vi "S4GUI.vi"(7 "Tab ObsEng":enum32{"Obs", "CCD modes", "Guider", "Eng"}(tab)) -> ()   [LabVIEW 2018] (continued)
            n4203 = call "Read WPROT.vi"("error in (no error)"=w9679, "Instrument in"=w9681) -> ("error out"=w9674:errorcluster, "Opt_Selector.lvclass"=w9677:refnum<class "Opt_Selector.lvclass">, "Instrument out"=w9682:refnum<class "Instrument.lvclass">)  [unwired: 7 in]
            n4204 = call-dynamic "Read sequencia_ant.vi"("error in (no error)"=w9674, "Opt_Selector in"=w9677) -> ("error out"=w9673:errorcluster, "sequencia_ant"=w9675:u16, "Opt_Selector out"=w9676:refnum<class "Opt_Selector.lvclass">)  [unwired: 7 in]
            n4205 = call-dynamic "Write sequencia.vi"("error in (no error)"=w9673, "sequencia"=w9675, "Opt_Selector in"=w9676) -> ("error out"=w9668:errorcluster, "Opt_Selector out"=w9669:refnum<class "Opt_Selector.lvclass">)  [unwired: 7 in]
            n4206 = call-dynamic "Read State Machine.vi"("error in (no error)"=w9668, "Device in"=w9669) -> ("error out"=w9671:errorcluster, "State Machine.lvclass"=w9666:refnum<class "State Machine.lvclass">, "Device out"=w9667:refnum<class "Opt_Selector.lvclass">)  [unwired: 7 in]
            n4207 = call "Next State.vi"("error in (no error)"=w9671, "New_State"=10, "State Machine in"=w9666) -> ("error out"=w9670:errorcluster, "State Machine out"=w9665:refnum<class "State Machine.lvclass">)  [unwired: 7 in]
            n4208 = call-dynamic "Write State Machine.vi"("error in (no error)"=w9670, "State Machine.lvclass"=w9665, "Device in"=w9667) -> ("error out"=w9664:errorcluster, "Device out"=w9663:refnum<class "Opt_Selector.lvclass">)  [unwired: 7 in]
            n4209 = call "Write WPROT.vi"("error in (no error)"=w9664, "Opt_Selector.lvclass"=w9663, "Instrument in"=w9682) -> ("error out"=w9661:errorcluster, "Instrument out"=w9662:refnum<class "Instrument.lvclass">)  [unwired: 7 in]
            n4210 = call "Write Instrument.lvclass.vi"("error in (no error)"=w9661, "Instrument.lvclass"=w9662, "S4ACS_GUI in"=w9680) -> ("error out"=w9683:errorcluster, "S4ACS_GUI out"=w9684:refnum<class "S4GUI.lvclass">)  [unwired: 7 in]
            n4211 = call-dynamic "Write ciclos.vi"("error in (no error)"=w9683, "ciclos"=u32 0, "S4ACS_GUI in"=w9684) -> ("error out"=w9657:errorcluster, "S4ACS_GUI out"=w9658:refnum<class "S4GUI.lvclass">)  [unwired: 7 in]
          }
          frame Enabled {
            w9774 = FALSE ("Wait Until Done")
            n4212 = call <vilib>:"Application Directory.vi"() -> ("Application Directory"=w9769:path)
            n4213 = Build Path(base path=w9769, name or relative path="MsgAbortSync.vi") -> (appended path=w9777:path)
            n4214 = Open VI Reference(vi path=w9777, error in (no error)=w9772) -> (vi reference=w9776:refnum<vi>, error out=w9775:errorcluster)  [unwired: 4 in]
            n4215 = invoke class="VI" method="Run VI"(reference=w9776, error in=w9775, "Wait until done"=w9774, "Auto Dispose Ref"=w9774) -> (error out=w9771:errorcluster)  [unwired: 1 in, 4 out]
          }
        }
        n4216 = property on="#Cycles Done" class="Slide (strict)"(error in=w9653, "Scale.Maximum"=w9655, "Scale.Minimum"=w9655) -> (error out=w9656:errorcluster)  [unwired: 1 in, 1 out]
      }
      event "Pause SM": Value Change {
        n4217 = event-data() -> ()  [unwired: 1 in, 6 out]
        n4218 = call-dynamic "Write User Event.vi"("error in (no error)"=w9781, "User Event"="PAUSE SM CLICKED", "S4GUI in"=w9782) -> ("error out"=w9779:errorcluster, "S4GUI out"=w9780:refnum<class "S4GUI.lvclass">)  [unwired: 7 in]
        n4219 = disable-structure shown="Enabled" {
          disable-tunnel: w9780 -> [w9796 w9806]
          disable-tunnel: w9779 -> [w9795 w9807]
          disable-tunnel: [w9786 w9806] -> w9784
          disable-tunnel: [w9785 w9805] -> w9783
          frame Disabled {
            n4220 = disable-structure shown="Enabled" {
              disable-tunnel: w9796 -> [w9800 w9803]
              disable-tunnel: w9795 -> [w9799 w9802]
              disable-tunnel: [w9798 w9803] -> w9789
              disable-tunnel: [w9797 w9802] -> w9788
              frame Disabled {
                n4221 = call-dynamic "Write paused.vi"("error in (no error)"=w9799, "paused"=TRUE ("stopped"), "S4ACS_GUI in"=w9800) -> ("error out"=w9797:errorcluster, "S4ACS_GUI out"=w9798:refnum<class "S4GUI.lvclass">)  [unwired: 7 in]
              }
              frame Enabled {
              }
            }
            n4222 = call-dynamic "Read Obs_state.vi"("error in (no error)"=w9788, "S4ACS_GUI in"=w9789) -> ("error out"=w9792:errorcluster, "Obs_state"=w9794:u32, "S4ACS_GUI out"=w9793:refnum<class "S4GUI.lvclass">)  [unwired: 7 in]
            n4223 = call-dynamic "Write Obs_prevstate.vi"("error in (no error)"=w9792, "Obs_prevstate"=w9794, "S4ACS_GUI in"=w9793) -> ("error out"=w9790:errorcluster, "S4ACS_GUI out"=w9791:refnum<class "S4GUI.lvclass">)  [unwired: 7 in]
            n4224 = call-dynamic "Write Obs_state.vi"("error in (no error)"=w9790, "Obs_state"=u32 400, "S4ACS_GUI in"=w9791) -> ("error out"=w9785:errorcluster, "S4ACS_GUI out"=w9786:refnum<class "S4GUI.lvclass">)  [unwired: 7 in]
          }
          frame Enabled {
            w9809 = FALSE ("Wait Until Done")
            n4225 = call <vilib>:"Application Directory.vi"() -> ("Application Directory"=w9804:path)
            n4226 = Build Path(base path=w9804, name or relative path="MsgPauseSync.vi") -> (appended path=w9812:path)
            n4227 = Open VI Reference(vi path=w9812, error in (no error)=w9807) -> (vi reference=w9811:refnum<vi>, error out=w9810:errorcluster)  [unwired: 4 in]
            n4228 = invoke class="VI" method="Run VI"(reference=w9811, error in=w9810, "Wait until done"=w9809, "Auto Dispose Ref"=w9809) -> (error out=w9805:errorcluster)  [unwired: 1 in, 4 out]
          }
        }
      }
      event "Abort ch1": Value Change {
        n4229 = event-data() -> ()  [unwired: 1 in, 6 out]
        n4230 = disable-structure shown="Enabled" {
          disable-tunnel: w9816 -> [w9849 w9871]
          disable-tunnel: w9815 -> [w9847 w9865]
          disable-tunnel: [w9829 w9864] -> w9814
          disable-tunnel: [w9817 w9871] -> w9813
          frame Disabled {
            # "Para movimento \nda lamina retardadora"
            # "Restaura a última sequência de lâminas"
            n4231 = call-dynamic "Read AcquisitionA.vi"("error in (no error)"=w9847, "S4ACS_GUI in"=w9849) -> ("error out"=w9852:errorcluster, "Acquisition.lvclass"=w9851:refnum<class "Acquisition.lvclass">, "S4ACS_GUI out"=w9848:refnum<class "S4GUI.lvclass">)  [unwired: 7 in]
            n4232 = call-dynamic "Read Channel.vi"("error in (no error)"=w9852, "Acquisition in"=w9851) -> ("error out"=w9854:errorcluster, "Channel.lvclass"=w9853:refnum<class "Channel.lvclass">, "Acquisition out"=w9860:refnum<class "Acquisition.lvclass">)  [unwired: 7 in]
            n4233 = call-dynamic "Read State Machine.vi"("error in (no error)"=w9854, "Device in"=w9853) -> ("error out"=w9856:errorcluster, "State Machine.lvclass"=w9855:refnum<class "State Machine.lvclass">, "Device out"=w9858:refnum<class "Channel.lvclass">)  [unwired: 7 in]
            n4234 = call "Next State.vi"("error in (no error)"=w9856, "New_State"=u32 80, "State Machine in"=w9855) -> ("error out"=w9859:errorcluster, "State Machine out"=w9857:refnum<class "State Machine.lvclass">)  [unwired: 7 in]
            n4235 = call-dynamic "Write State Machine.vi"("error in (no error)"=w9859, "State Machine.lvclass"=w9857, "Device in"=w9858) -> ("error out"=w9861:errorcluster, "Device out"=w9862:refnum<class "Channel.lvclass">)  [unwired: 7 in]
            n4236 = call-dynamic "Write Channel.vi"("error in (no error)"=w9861, "Channel.lvclass"=w9862, "Acquisition in"=w9860) -> ("error out"=w9844:errorcluster, "Acquisition out"=w9845:refnum<class "Acquisition.lvclass">)  [unwired: 7 in]
            n4237 = call-dynamic "Write Acq_state.vi"("error in (no error)"=w9844, "Acq_state"=u32 0, "Acquisition in"=w9845) -> ("error out"=w9843:errorcluster, "Acquisition out"=w9842:refnum<class "Acquisition.lvclass">)  [unwired: 7 in]
            n4238 = call-dynamic "Write AcquisitionA.vi"("error in (no error)"=w9843, "Acquisition.lvclass"=w9842, "S4ACS_GUI in"=w9848) -> ("error out"=w9830:errorcluster, "S4ACS_GUI out"=w9828:refnum<class "S4GUI.lvclass">)  [unwired: 7 in]
            n4239 = call "Read Instrument.lvclass.vi"("error in (no error)"=w9830, "S4ACS_GUI in"=w9828) -> ("error out"=w9837:errorcluster, "Instrument.lvclass"=w9840:refnum<class "Instrument.lvclass">, "S4ACS_GUI out"=w9841:refnum<class "S4GUI.lvclass">)  [unwired: 7 in]
            n4240 = call "Read WPROT.vi"("error in (no error)"=w9837, "Instrument in"=w9840) -> ("error out"=w9836:errorcluster, "Opt_Selector.lvclass"=w9838:refnum<class "Opt_Selector.lvclass">, "Instrument out"=w9839:refnum<class "Instrument.lvclass">)  [unwired: 7 in]
            n4241 = call-dynamic "Read sequencia_ant.vi"("error in (no error)"=w9836, "Opt_Selector in"=w9838) -> ("error out"=w9832:errorcluster, "sequencia_ant"=w9831:u16, "Opt_Selector out"=w9833:refnum<class "Opt_Selector.lvclass">)  [unwired: 7 in]
            n4242 = call-dynamic "Write sequencia.vi"("error in (no error)"=w9832, "sequencia"=w9831, "Opt_Selector in"=w9833) -> ("error out"=w9821:errorcluster, "Opt_Selector out"=w9822:refnum<class "Opt_Selector.lvclass">)  [unwired: 7 in]
            n4243 = call-dynamic "Read State Machine.vi"("error in (no error)"=w9821, "Device in"=w9822) -> ("error out"=w9824:errorcluster, "State Machine.lvclass"=w9827:refnum<class "State Machine.lvclass">, "Device out"=w9820:refnum<class "Opt_Selector.lvclass">)  [unwired: 7 in]
            n4244 = call "Next State.vi"("error in (no error)"=w9824, "New_State"=10, "State Machine in"=w9827) -> ("error out"=w9823:errorcluster, "State Machine out"=w9826:refnum<class "State Machine.lvclass">)  [unwired: 7 in]
            n4245 = call-dynamic "Write State Machine.vi"("error in (no error)"=w9823, "State Machine.lvclass"=w9826, "Device in"=w9820) -> ("error out"=w9818:errorcluster, "Device out"=w9819:refnum<class "Opt_Selector.lvclass">)  [unwired: 7 in]
            n4246 = call "Write WPROT.vi"("error in (no error)"=w9818, "Opt_Selector.lvclass"=w9819, "Instrument in"=w9839) -> ("error out"=w9835:errorcluster, "Instrument out"=w9834:refnum<class "Instrument.lvclass">)  [unwired: 7 in]
            n4247 = call "Write Instrument.lvclass.vi"("error in (no error)"=w9835, "Instrument.lvclass"=w9834, "S4ACS_GUI in"=w9841) -> ("error out"=w9829:errorcluster, "S4ACS_GUI out"=w9817:refnum<class "S4GUI.lvclass">)  [unwired: 7 in]
          }
          frame Enabled {
            w9867 = FALSE ("Wait Until Done")
            n4248 = call <vilib>:"Application Directory.vi"() -> ("Application Directory"=w9863:path)
            n4249 = Build Path(base path=w9863, name or relative path="MsgAbort1.vi") -> (appended path=w9870:path)
            n4250 = Open VI Reference(vi path=w9870, error in (no error)=w9865) -> (vi reference=w9869:refnum<vi>, error out=w9868:errorcluster)  [unwired: 4 in]
            n4251 = invoke class="VI" method="Run VI"(reference=w9869, error in=w9868, "Wait until done"=w9867, "Auto Dispose Ref"=w9867) -> (error out=w9864:errorcluster)  [unwired: 1 in, 4 out]
          }
        }
      }
      event "Abort ch2": Value Change {
        n4252 = event-data() -> ()  [unwired: 1 in, 6 out]
        n4253 = disable-structure shown="Enabled" {
          disable-tunnel: w9875 -> [w9908 w9924]
          disable-tunnel: w9874 -> [w9906 w9925]
          disable-tunnel: [w9888 w9923] -> w9873
          disable-tunnel: [w9876 w9924] -> w9872
          frame Disabled {
            # "Para movimento \nda lamina retardadora"
            # "Restaura a última sequência de lâminas"
            n4254 = call "Read AcquisitionB.vi"("error in (no error)"=w9906, "S4ACS_GUI in"=w9908) -> ("error out"=w9911:errorcluster, "Acquisition.lvclass"=w9910:refnum<class "Acquisition.lvclass">, "S4ACS_GUI out"=w9907:refnum<class "S4GUI.lvclass">)  [unwired: 7 in]
            n4255 = call-dynamic "Read Channel.vi"("error in (no error)"=w9911, "Acquisition in"=w9910) -> ("error out"=w9913:errorcluster, "Channel.lvclass"=w9912:refnum<class "Channel.lvclass">, "Acquisition out"=w9919:refnum<class "Acquisition.lvclass">)  [unwired: 7 in]
            n4256 = call-dynamic "Read State Machine.vi"("error in (no error)"=w9913, "Device in"=w9912) -> ("error out"=w9915:errorcluster, "State Machine.lvclass"=w9914:refnum<class "State Machine.lvclass">, "Device out"=w9917:refnum<class "Channel.lvclass">)  [unwired: 7 in]
            n4257 = call "Next State.vi"("error in (no error)"=w9915, "New_State"=u32 80, "State Machine in"=w9914) -> ("error out"=w9918:errorcluster, "State Machine out"=w9916:refnum<class "State Machine.lvclass">)  [unwired: 7 in]
            n4258 = call-dynamic "Write State Machine.vi"("error in (no error)"=w9918, "State Machine.lvclass"=w9916, "Device in"=w9917) -> ("error out"=w9920:errorcluster, "Device out"=w9921:refnum<class "Channel.lvclass">)  [unwired: 7 in]
            n4259 = call-dynamic "Write Channel.vi"("error in (no error)"=w9920, "Channel.lvclass"=w9921, "Acquisition in"=w9919) -> ("error out"=w9903:errorcluster, "Acquisition out"=w9904:refnum<class "Acquisition.lvclass">)  [unwired: 7 in]
            n4260 = call-dynamic "Write Acq_state.vi"("error in (no error)"=w9903, "Acq_state"=u32 0, "Acquisition in"=w9904) -> ("error out"=w9902:errorcluster, "Acquisition out"=w9901:refnum<class "Acquisition.lvclass">)  [unwired: 7 in]
            n4261 = call "Write AcquisitionB.vi"("error in (no error)"=w9902, "Acquisition.lvclass"=w9901, "S4ACS_GUI in"=w9907) -> ("error out"=w9889:errorcluster, "S4ACS_GUI out"=w9887:refnum<class "S4GUI.lvclass">)  [unwired: 7 in]
            n4262 = call "Read Instrument.lvclass.vi"("error in (no error)"=w9889, "S4ACS_GUI in"=w9887) -> ("error out"=w9896:errorcluster, "Instrument.lvclass"=w9899:refnum<class "Instrument.lvclass">, "S4ACS_GUI out"=w9900:refnum<class "S4GUI.lvclass">)  [unwired: 7 in]
            n4263 = call "Read WPROT.vi"("error in (no error)"=w9896, "Instrument in"=w9899) -> ("error out"=w9895:errorcluster, "Opt_Selector.lvclass"=w9897:refnum<class "Opt_Selector.lvclass">, "Instrument out"=w9898:refnum<class "Instrument.lvclass">)  [unwired: 7 in]
            n4264 = call-dynamic "Read sequencia_ant.vi"("error in (no error)"=w9895, "Opt_Selector in"=w9897) -> ("error out"=w9891:errorcluster, "sequencia_ant"=w9890:u16, "Opt_Selector out"=w9892:refnum<class "Opt_Selector.lvclass">)  [unwired: 7 in]
            n4265 = call-dynamic "Write sequencia.vi"("error in (no error)"=w9891, "sequencia"=w9890, "Opt_Selector in"=w9892) -> ("error out"=w9880:errorcluster, "Opt_Selector out"=w9881:refnum<class "Opt_Selector.lvclass">)  [unwired: 7 in]
            n4266 = call-dynamic "Read State Machine.vi"("error in (no error)"=w9880, "Device in"=w9881) -> ("error out"=w9883:errorcluster, "State Machine.lvclass"=w9886:refnum<class "State Machine.lvclass">, "Device out"=w9879:refnum<class "Opt_Selector.lvclass">)  [unwired: 7 in]
            n4267 = call "Next State.vi"("error in (no error)"=w9883, "New_State"=10, "State Machine in"=w9886) -> ("error out"=w9882:errorcluster, "State Machine out"=w9885:refnum<class "State Machine.lvclass">)  [unwired: 7 in]
            n4268 = call-dynamic "Write State Machine.vi"("error in (no error)"=w9882, "State Machine.lvclass"=w9885, "Device in"=w9879) -> ("error out"=w9877:errorcluster, "Device out"=w9878:refnum<class "Opt_Selector.lvclass">)  [unwired: 7 in]
            n4269 = call "Write WPROT.vi"("error in (no error)"=w9877, "Opt_Selector.lvclass"=w9878, "Instrument in"=w9898) -> ("error out"=w9894:errorcluster, "Instrument out"=w9893:refnum<class "Instrument.lvclass">)  [unwired: 7 in]
            n4270 = call "Write Instrument.lvclass.vi"("error in (no error)"=w9894, "Instrument.lvclass"=w9893, "S4ACS_GUI in"=w9900) -> ("error out"=w9888:errorcluster, "S4ACS_GUI out"=w9876:refnum<class "S4GUI.lvclass">)  [unwired: 7 in]
          }
          frame Enabled {
            w9927 = FALSE ("Wait Until Done")
            n4271 = call <vilib>:"Application Directory.vi"() -> ("Application Directory"=w9922:path)
            n4272 = Build Path(base path=w9922, name or relative path="MsgAbort2.vi") -> (appended path=w9930:path)
            n4273 = Open VI Reference(vi path=w9930, error in (no error)=w9925) -> (vi reference=w9929:refnum<vi>, error out=w9928:errorcluster)  [unwired: 4 in]
            n4274 = invoke class="VI" method="Run VI"(reference=w9929, error in=w9928, "Wait until done"=w9927, "Auto Dispose Ref"=w9927) -> (error out=w9923:errorcluster)  [unwired: 1 in, 4 out]
          }
        }
      }
      event "Abort ch3": Value Change {
        n4275 = event-data() -> ()  [unwired: 1 in, 6 out]
        n4276 = disable-structure shown="Enabled" {
          disable-tunnel: w9934 -> [w9967 w9983]
          disable-tunnel: w9933 -> [w9965 w9984]
          disable-tunnel: [w9947 w9982] -> w9932
          disable-tunnel: [w9935 w9983] -> w9931
          frame Disabled {
            # "Para movimento \nda lamina retardadora"
            # "Restaura a última sequência de lâminas"
            n4277 = call-dynamic "Read AcquisitionC.vi"("error in (no error)"=w9965, "S4ACS_GUI in"=w9967) -> ("error out"=w9970:errorcluster, "Acquisition.lvclass"=w9969:refnum<class "Acquisition.lvclass">, "S4ACS_GUI out"=w9966:refnum<class "S4GUI.lvclass">)  [unwired: 7 in]
            n4278 = call-dynamic "Read Channel.vi"("error in (no error)"=w9970, "Acquisition in"=w9969) -> ("error out"=w9972:errorcluster, "Channel.lvclass"=w9971:refnum<class "Channel.lvclass">, "Acquisition out"=w9978:refnum<class "Acquisition.lvclass">)  [unwired: 7 in]
            n4279 = call-dynamic "Read State Machine.vi"("error in (no error)"=w9972, "Device in"=w9971) -> ("error out"=w9974:errorcluster, "State Machine.lvclass"=w9973:refnum<class "State Machine.lvclass">, "Device out"=w9976:refnum<class "Channel.lvclass">)  [unwired: 7 in]
            n4280 = call "Next State.vi"("error in (no error)"=w9974, "New_State"=u32 80, "State Machine in"=w9973) -> ("error out"=w9977:errorcluster, "State Machine out"=w9975:refnum<class "State Machine.lvclass">)  [unwired: 7 in]
            n4281 = call-dynamic "Write State Machine.vi"("error in (no error)"=w9977, "State Machine.lvclass"=w9975, "Device in"=w9976) -> ("error out"=w9979:errorcluster, "Device out"=w9980:refnum<class "Channel.lvclass">)  [unwired: 7 in]
            n4282 = call-dynamic "Write Channel.vi"("error in (no error)"=w9979, "Channel.lvclass"=w9980, "Acquisition in"=w9978) -> ("error out"=w9962:errorcluster, "Acquisition out"=w9963:refnum<class "Acquisition.lvclass">)  [unwired: 7 in]
            n4283 = call-dynamic "Write Acq_state.vi"("error in (no error)"=w9962, "Acq_state"=u32 0, "Acquisition in"=w9963) -> ("error out"=w9961:errorcluster, "Acquisition out"=w9960:refnum<class "Acquisition.lvclass">)  [unwired: 7 in]
            n4284 = call-dynamic "Write AcquisitionC.vi"("error in (no error)"=w9961, "Acquisition.lvclass"=w9960, "S4ACS_GUI in"=w9966) -> ("error out"=w9948:errorcluster, "S4ACS_GUI out"=w9946:refnum<class "S4GUI.lvclass">)  [unwired: 7 in]
            n4285 = call "Read Instrument.lvclass.vi"("error in (no error)"=w9948, "S4ACS_GUI in"=w9946) -> ("error out"=w9955:errorcluster, "Instrument.lvclass"=w9958:refnum<class "Instrument.lvclass">, "S4ACS_GUI out"=w9959:refnum<class "S4GUI.lvclass">)  [unwired: 7 in]
            n4286 = call "Read WPROT.vi"("error in (no error)"=w9955, "Instrument in"=w9958) -> ("error out"=w9954:errorcluster, "Opt_Selector.lvclass"=w9956:refnum<class "Opt_Selector.lvclass">, "Instrument out"=w9957:refnum<class "Instrument.lvclass">)  [unwired: 7 in]
            n4287 = call-dynamic "Read sequencia_ant.vi"("error in (no error)"=w9954, "Opt_Selector in"=w9956) -> ("error out"=w9950:errorcluster, "sequencia_ant"=w9949:u16, "Opt_Selector out"=w9951:refnum<class "Opt_Selector.lvclass">)  [unwired: 7 in]
            n4288 = call-dynamic "Write sequencia.vi"("error in (no error)"=w9950, "sequencia"=w9949, "Opt_Selector in"=w9951) -> ("error out"=w9939:errorcluster, "Opt_Selector out"=w9940:refnum<class "Opt_Selector.lvclass">)  [unwired: 7 in]
            n4289 = call-dynamic "Read State Machine.vi"("error in (no error)"=w9939, "Device in"=w9940) -> ("error out"=w9942:errorcluster, "State Machine.lvclass"=w9945:refnum<class "State Machine.lvclass">, "Device out"=w9938:refnum<class "Opt_Selector.lvclass">)  [unwired: 7 in]
            n4290 = call "Next State.vi"("error in (no error)"=w9942, "New_State"=10, "State Machine in"=w9945) -> ("error out"=w9941:errorcluster, "State Machine out"=w9944:refnum<class "State Machine.lvclass">)  [unwired: 7 in]
            n4291 = call-dynamic "Write State Machine.vi"("error in (no error)"=w9941, "State Machine.lvclass"=w9944, "Device in"=w9938) -> ("error out"=w9936:errorcluster, "Device out"=w9937:refnum<class "Opt_Selector.lvclass">)  [unwired: 7 in]
            n4292 = call "Write WPROT.vi"("error in (no error)"=w9936, "Opt_Selector.lvclass"=w9937, "Instrument in"=w9957) -> ("error out"=w9953:errorcluster, "Instrument out"=w9952:refnum<class "Instrument.lvclass">)  [unwired: 7 in]
            n4293 = call "Write Instrument.lvclass.vi"("error in (no error)"=w9953, "Instrument.lvclass"=w9952, "S4ACS_GUI in"=w9959) -> ("error out"=w9947:errorcluster, "S4ACS_GUI out"=w9935:refnum<class "S4GUI.lvclass">)  [unwired: 7 in]
          }
          frame Enabled {
            w9986 = FALSE ("Wait Until Done")
            n4294 = call <vilib>:"Application Directory.vi"() -> ("Application Directory"=w9981:path)
            n4295 = Build Path(base path=w9981, name or relative path="MsgAbort3.vi") -> (appended path=w9989:path)
            n4296 = Open VI Reference(vi path=w9989, error in (no error)=w9984) -> (vi reference=w9988:refnum<vi>, error out=w9987:errorcluster)  [unwired: 4 in]
            n4297 = invoke class="VI" method="Run VI"(reference=w9988, error in=w9987, "Wait until done"=w9986, "Auto Dispose Ref"=w9986) -> (error out=w9982:errorcluster)  [unwired: 1 in, 4 out]
          }
        }
      }
      event "Abort ch4": Value Change {
        n4298 = event-data() -> ()  [unwired: 1 in, 6 out]
        n4299 = disable-structure shown="Enabled" {
          disable-tunnel: w9993 -> [w10026 w10042]
          disable-tunnel: w9992 -> [w10024 w10043]
          disable-tunnel: [w10006 w10041] -> w9991
          disable-tunnel: [w9994 w10042] -> w9990
          frame Disabled {
            # "Para movimento \nda lamina retardadora"
            # "Restaura a última sequência de lâminas"
            n4300 = call-dynamic "Read AcquisitionD.vi"("error in (no error)"=w10024, "S4ACS_GUI in"=w10026) -> ("error out"=w10029:errorcluster, "Acquisition.lvclass"=w10028:refnum<class "Acquisition.lvclass">, "S4ACS_GUI out"=w10025:refnum<class "S4GUI.lvclass">)  [unwired: 7 in]
            n4301 = call-dynamic "Read Channel.vi"("error in (no error)"=w10029, "Acquisition in"=w10028) -> ("error out"=w10031:errorcluster, "Channel.lvclass"=w10030:refnum<class "Channel.lvclass">, "Acquisition out"=w10037:refnum<class "Acquisition.lvclass">)  [unwired: 7 in]
            n4302 = call-dynamic "Read State Machine.vi"("error in (no error)"=w10031, "Device in"=w10030) -> ("error out"=w10033:errorcluster, "State Machine.lvclass"=w10032:refnum<class "State Machine.lvclass">, "Device out"=w10035:refnum<class "Channel.lvclass">)  [unwired: 7 in]
            n4303 = call "Next State.vi"("error in (no error)"=w10033, "New_State"=u32 80, "State Machine in"=w10032) -> ("error out"=w10036:errorcluster, "State Machine out"=w10034:refnum<class "State Machine.lvclass">)  [unwired: 7 in]
            n4304 = call-dynamic "Write State Machine.vi"("error in (no error)"=w10036, "State Machine.lvclass"=w10034, "Device in"=w10035) -> ("error out"=w10038:errorcluster, "Device out"=w10039:refnum<class "Channel.lvclass">)  [unwired: 7 in]
            n4305 = call-dynamic "Write Channel.vi"("error in (no error)"=w10038, "Channel.lvclass"=w10039, "Acquisition in"=w10037) -> ("error out"=w10021:errorcluster, "Acquisition out"=w10022:refnum<class "Acquisition.lvclass">)  [unwired: 7 in]
            n4306 = call-dynamic "Write Acq_state.vi"("error in (no error)"=w10021, "Acq_state"=u32 0, "Acquisition in"=w10022) -> ("error out"=w10020:errorcluster, "Acquisition out"=w10019:refnum<class "Acquisition.lvclass">)  [unwired: 7 in]
            n4307 = call-dynamic "Write AcquisitionD.vi"("error in (no error)"=w10020, "Acquisition.lvclass"=w10019, "S4ACS_GUI in"=w10025) -> ("error out"=w10007:errorcluster, "S4ACS_GUI out"=w10005:refnum<class "S4GUI.lvclass">)  [unwired: 7 in]
            n4308 = call "Read Instrument.lvclass.vi"("error in (no error)"=w10007, "S4ACS_GUI in"=w10005) -> ("error out"=w10014:errorcluster, "Instrument.lvclass"=w10017:refnum<class "Instrument.lvclass">, "S4ACS_GUI out"=w10018:refnum<class "S4GUI.lvclass">)  [unwired: 7 in]
            n4309 = call "Read WPROT.vi"("error in (no error)"=w10014, "Instrument in"=w10017) -> ("error out"=w10013:errorcluster, "Opt_Selector.lvclass"=w10015:refnum<class "Opt_Selector.lvclass">, "Instrument out"=w10016:refnum<class "Instrument.lvclass">)  [unwired: 7 in]
            n4310 = call-dynamic "Read sequencia_ant.vi"("error in (no error)"=w10013, "Opt_Selector in"=w10015) -> ("error out"=w10009:errorcluster, "sequencia_ant"=w10008:u16, "Opt_Selector out"=w10010:refnum<class "Opt_Selector.lvclass">)  [unwired: 7 in]
            n4311 = call-dynamic "Write sequencia.vi"("error in (no error)"=w10009, "sequencia"=w10008, "Opt_Selector in"=w10010) -> ("error out"=w9998:errorcluster, "Opt_Selector out"=w9999:refnum<class "Opt_Selector.lvclass">)  [unwired: 7 in]
            n4312 = call-dynamic "Read State Machine.vi"("error in (no error)"=w9998, "Device in"=w9999) -> ("error out"=w10001:errorcluster, "State Machine.lvclass"=w10004:refnum<class "State Machine.lvclass">, "Device out"=w9997:refnum<class "Opt_Selector.lvclass">)  [unwired: 7 in]
            n4313 = call "Next State.vi"("error in (no error)"=w10001, "New_State"=10, "State Machine in"=w10004) -> ("error out"=w10000:errorcluster, "State Machine out"=w10003:refnum<class "State Machine.lvclass">)  [unwired: 7 in]
            n4314 = call-dynamic "Write State Machine.vi"("error in (no error)"=w10000, "State Machine.lvclass"=w10003, "Device in"=w9997) -> ("error out"=w9995:errorcluster, "Device out"=w9996:refnum<class "Opt_Selector.lvclass">)  [unwired: 7 in]
            n4315 = call "Write WPROT.vi"("error in (no error)"=w9995, "Opt_Selector.lvclass"=w9996, "Instrument in"=w10016) -> ("error out"=w10012:errorcluster, "Instrument out"=w10011:refnum<class "Instrument.lvclass">)  [unwired: 7 in]
            n4316 = call "Write Instrument.lvclass.vi"("error in (no error)"=w10012, "Instrument.lvclass"=w10011, "S4ACS_GUI in"=w10018) -> ("error out"=w10006:errorcluster, "S4ACS_GUI out"=w9994:refnum<class "S4GUI.lvclass">)  [unwired: 7 in]
          }
          frame Enabled {
            w10045 = FALSE ("Wait Until Done")
            n4317 = call <vilib>:"Application Directory.vi"() -> ("Application Directory"=w10040:path)
            n4318 = Build Path(base path=w10040, name or relative path="MsgAbort4.vi") -> (appended path=w10048:path)
            n4319 = Open VI Reference(vi path=w10048, error in (no error)=w10043) -> (vi reference=w10047:refnum<vi>, error out=w10046:errorcluster)  [unwired: 4 in]
            n4320 = invoke class="VI" method="Run VI"(reference=w10047, error in=w10046, "Wait until done"=w10045, "Auto Dispose Ref"=w10045) -> (error out=w10041:errorcluster)  [unwired: 1 in, 4 out]
          }
        }
      }
      event "SyncBox": Value Change {
        n4321 = event-data() -> ()  [unwired: 1 in, 4 out]
        n4322 = call-dynamic "Read Sync Box.lvclass.vi"("error in (no error)"=w10051, "SPARC4_AC in"=w10052) -> ("error out"=w10067:errorcluster, "Sync Box.lvclass"=w10068:refnum<class "Sync Box.lvclass">, "SPARC4_AC out"=w10056:refnum<class "S4GUI.lvclass">)  [unwired: 7 in]
        n4323 = call-dynamic "Read Trigger.lvclass.vi"("error in (no error)"=w10067, "Sync Box in"=w10068) -> ("error out"=w10065:errorcluster, "Trigger.lvclass"=w10066:refnum<class "Trigger.lvclass">, "Sync Box out"=w10059:refnum<class "Sync Box.lvclass">)  [unwired: 7 in]
        n4324 = call-dynamic "Read State Machine.vi"("error in (no error)"=w10065, "Device in"=w10066) -> ("error out"=w10063:errorcluster, "State Machine.lvclass"=w10064:refnum<class "State Machine.lvclass">, "Device out"=w10060:refnum<class "Trigger.lvclass">)  [unwired: 7 in]
        n4325 = call "Next State.vi"("error in (no error)"=w10063, "New_State"=u32 1, "State Machine in"=w10064) -> ("error out"=w10058:errorcluster, "State Machine out"=w10061:refnum<class "State Machine.lvclass">)  [unwired: 7 in]
        n4326 = call-dynamic "Write State Machine.vi"("error in (no error)"=w10058, "State Machine.lvclass"=w10061, "Device in"=w10060) -> ("error out"=w10054:errorcluster, "Device out"=w10053:refnum<class "Trigger.lvclass">)  [unwired: 7 in]
        n4327 = call-dynamic "Write Trigger.lvclass.vi"("error in (no error)"=w10054, "Trigger.lvclass"=w10053, "Sync Box in"=w10059) -> ("error out"=w10055:errorcluster, "Sync Box out"=w10057:refnum<class "Sync Box.lvclass">)  [unwired: 7 in]
        n4328 = call-dynamic "Write Sync Box.lvclass.vi"("error in (no error)"=w10055, "Sync Box.lvclass"=w10057, "SPARC4_AC in"=w10056) -> ("error out"=w10050:errorcluster, "SPARC4_AC out"=w10049:refnum<class "S4GUI.lvclass">)  [unwired: 7 in]
      }
      event "Fire manual", "Fire": Value Change {
        n4329 = event-data() -> ()  [unwired: 1 in, 4 out]
        n4330 = call-dynamic "Read Sync Box.lvclass.vi"("error in (no error)"=w10071, "SPARC4_AC in"=w10072) -> ("error out"=w10087:errorcluster, "Sync Box.lvclass"=w10088:refnum<class "Sync Box.lvclass">, "SPARC4_AC out"=w10076:refnum<class "S4GUI.lvclass">)  [unwired: 7 in]
        n4331 = call-dynamic "Read Trigger.lvclass.vi"("error in (no error)"=w10087, "Sync Box in"=w10088) -> ("error out"=w10085:errorcluster, "Trigger.lvclass"=w10086:refnum<class "Trigger.lvclass">, "Sync Box out"=w10079:refnum<class "Sync Box.lvclass">)  [unwired: 7 in]
        n4332 = call-dynamic "Read State Machine.vi"("error in (no error)"=w10085, "Device in"=w10086) -> ("error out"=w10083:errorcluster, "State Machine.lvclass"=w10084:refnum<class "State Machine.lvclass">, "Device out"=w10080:refnum<class "Trigger.lvclass">)  [unwired: 7 in]
        n4333 = call "Next State.vi"("error in (no error)"=w10083, "New_State"=u32 40, "State Machine in"=w10084) -> ("error out"=w10078:errorcluster, "State Machine out"=w10081:refnum<class "State Machine.lvclass">)  [unwired: 7 in]
        n4334 = call-dynamic "Write State Machine.vi"("error in (no error)"=w10078, "State Machine.lvclass"=w10081, "Device in"=w10080) -> ("error out"=w10074:errorcluster, "Device out"=w10073:refnum<class "Trigger.lvclass">)  [unwired: 7 in]
        n4335 = call-dynamic "Write Trigger.lvclass.vi"("error in (no error)"=w10074, "Trigger.lvclass"=w10073, "Sync Box in"=w10079) -> ("error out"=w10075:errorcluster, "Sync Box out"=w10077:refnum<class "Sync Box.lvclass">)  [unwired: 7 in]
        n4336 = call-dynamic "Write Sync Box.lvclass.vi"("error in (no error)"=w10075, "Sync Box.lvclass"=w10077, "SPARC4_AC in"=w10076) -> ("error out"=w10070:errorcluster, "SPARC4_AC out"=w10069:refnum<class "S4GUI.lvclass">)  [unwired: 7 in]
      }
      event "Select Trigger Mode": Value Change {
        n4337 = event-data() -> ("NewVal"=w10090:bool)  [unwired: 1 in, 2 out]
        n4338 = call-dynamic "Read Sync Box.lvclass.vi"("error in (no error)"=w10098, "SPARC4_AC in"=w10099) -> ("error out"=w10110:errorcluster, "Sync Box.lvclass"=w10111:refnum<class "Sync Box.lvclass">, "SPARC4_AC out"=w10103:refnum<class "S4GUI.lvclass">)  [unwired: 7 in]
        n4339 = call-dynamic "Read Trigger.lvclass.vi"("error in (no error)"=w10110, "Sync Box in"=w10111) -> ("error out"=w10091:errorcluster, "Trigger.lvclass"=w10094:refnum<class "Trigger.lvclass">, "Sync Box out"=w10106:refnum<class "Sync Box.lvclass">)  [unwired: 7 in]
        n4340 = call-dynamic "Write Trigger Mode Target.vi"("error in (no error)"=w10091, "Trigger Mode Target"=w10090, "Trigger in"=w10094) -> ("error out"=w10092:errorcluster, "Trigger out"=w10093:refnum<class "Trigger.lvclass">)  [unwired: 7 in]
        n4341 = call-dynamic "Read State Machine.vi"("error in (no error)"=w10092, "Device in"=w10093) -> ("error out"=w10095:errorcluster, "State Machine.lvclass"=w10096:refnum<class "State Machine.lvclass">, "Device out"=w10107:refnum<class "Trigger.lvclass">)  [unwired: 7 in]
        n4342 = call "Next State.vi"("error in (no error)"=w10095, "New_State"=u32 30, "State Machine in"=w10096) -> ("error out"=w10105:errorcluster, "State Machine out"=w10108:refnum<class "State Machine.lvclass">)  [unwired: 7 in]
        n4343 = call-dynamic "Write State Machine.vi"("error in (no error)"=w10105, "State Machine.lvclass"=w10108, "Device in"=w10107) -> ("error out"=w10101:errorcluster, "Device out"=w10100:refnum<class "Trigger.lvclass">)  [unwired: 7 in]
        n4344 = call-dynamic "Write Trigger.lvclass.vi"("error in (no error)"=w10101, "Trigger.lvclass"=w10100, "Sync Box in"=w10106) -> ("error out"=w10102:errorcluster, "Sync Box out"=w10104:refnum<class "Sync Box.lvclass">)  [unwired: 7 in]
        n4345 = call-dynamic "Write Sync Box.lvclass.vi"("error in (no error)"=w10102, "Sync Box.lvclass"=w10104, "SPARC4_AC in"=w10103) -> ("error out"=w10097:errorcluster, "SPARC4_AC out"=w10089:refnum<class "S4GUI.lvclass">)  [unwired: 7 in]
      }
      event "Set SyncBox": Value Change {
        n4346 = event-data() -> ()  [unwired: 1 in, 4 out]
        n4347 = call-dynamic "Read Sync Box.lvclass.vi"("error in (no error)"=w10114, "SPARC4_AC in"=w10115) -> ("error out"=w10130:errorcluster, "Sync Box.lvclass"=w10131:refnum<class "Sync Box.lvclass">, "SPARC4_AC out"=w10119:refnum<class "S4GUI.lvclass">)  [unwired: 7 in]
        n4348 = call-dynamic "Read Trigger.lvclass.vi"("error in (no error)"=w10130, "Sync Box in"=w10131) -> ("error out"=w10128:errorcluster, "Trigger.lvclass"=w10129:refnum<class "Trigger.lvclass">, "Sync Box out"=w10122:refnum<class "Sync Box.lvclass">)  [unwired: 7 in]
        n4349 = call-dynamic "Read State Machine.vi"("error in (no error)"=w10128, "Device in"=w10129) -> ("error out"=w10126:errorcluster, "State Machine.lvclass"=w10127:refnum<class "State Machine.lvclass">, "Device out"=w10123:refnum<class "Trigger.lvclass">)  [unwired: 7 in]
        n4350 = call "Next State.vi"("error in (no error)"=w10126, "New_State"=u32 10, "State Machine in"=w10127) -> ("error out"=w10121:errorcluster, "State Machine out"=w10124:refnum<class "State Machine.lvclass">)  [unwired: 7 in]
        n4351 = call-dynamic "Write State Machine.vi"("error in (no error)"=w10121, "State Machine.lvclass"=w10124, "Device in"=w10123) -> ("error out"=w10117:errorcluster, "Device out"=w10116:refnum<class "Trigger.lvclass">)  [unwired: 7 in]
        n4352 = call-dynamic "Write Trigger.lvclass.vi"("error in (no error)"=w10117, "Trigger.lvclass"=w10116, "Sync Box in"=w10122) -> ("error out"=w10118:errorcluster, "Sync Box out"=w10120:refnum<class "Sync Box.lvclass">)  [unwired: 7 in]
        n4353 = call-dynamic "Write Sync Box.lvclass.vi"("error in (no error)"=w10118, "Sync Box.lvclass"=w10120, "SPARC4_AC in"=w10119) -> ("error out"=w10113:errorcluster, "SPARC4_AC out"=w10112:refnum<class "S4GUI.lvclass">)  [unwired: 7 in]
      }
      event "Set Focus": Value Change {
        n4354 = event-data() -> ("NewVal"=w10132:bool)  [unwired: 1 in]
        n4355 = case shown="True" w10132 {
          tunnel: w10136 -> [w10138 w10147]
          tunnel: w10135 -> [w10137 w10146]
          tunnel: [w10137 w10145] -> w10134
          tunnel: [w10138 w10144] -> w10133
          frame False {
          }
          frame True {
            n4356 = call-dynamic "Read TelFocus.lvclass.vi"("error in (no error)"=w10146, "S4GUI in"=w10147) -> ("error out"=w10160:errorcluster, "TelFocus.lvclass"=w10161:refnum<class "TelFocus.lvclass">, "S4GUI out"=w10151:refnum<class "S4GUI.lvclass">)  [unwired: 7 in]
            n4357 = call-dynamic "Read SecMirror.lvclass.vi"("error in (no error)"=w10160, "TelFocus in"=w10161) -> ("error out"=w10140:errorcluster, "SecMirror.lvclass"=w10143:refnum<class "SecMirror.lvclass">, "TelFocus out"=w10154:refnum<class "TelFocus.lvclass">)  [unwired: 7 in]
            n4358 = call-dynamic "Write target.vi"("error in (no error)"=w10140, "target"="Target focus", "SecMirror in"=w10143) -> ("error out"=w10139:errorcluster, "SecMirror out"=w10142:refnum<class "SecMirror.lvclass">)  [unwired: 7 in]
            n4359 = call-dynamic "Read State Machine.vi"("error in (no error)"=w10139, "Device in"=w10142) -> ("error out"=w10158:errorcluster, "State Machine.lvclass"=w10159:refnum<class "State Machine.lvclass">, "Device out"=w10155:refnum<class "SecMirror.lvclass">)  [unwired: 7 in]
            n4360 = call "Next State.vi"("error in (no error)"=w10158, "New_State"=1, "State Machine in"=w10159) -> ("error out"=w10153:errorcluster, "State Machine out"=w10156:refnum<class "State Machine.lvclass">)  [unwired: 7 in]
            n4361 = call-dynamic "Write State Machine.vi"("error in (no error)"=w10153, "State Machine.lvclass"=w10156, "Device in"=w10155) -> ("error out"=w10149:errorcluster, "Device out"=w10148:refnum<class "SecMirror.lvclass">)  [unwired: 7 in]
            n4362 = call-dynamic "Write SecMirror.lvclass.vi"("error in (no error)"=w10149, "SecMirror.lvclass"=w10148, "TelFocus in"=w10154) -> ("error out"=w10150:errorcluster, "TelFocus out"=w10152:refnum<class "TelFocus.lvclass">)  [unwired: 7 in]
            n4363 = call-dynamic "Write TelFocus.lvclass.vi"("error in (no error)"=w10150, "TelFocus.lvclass"=w10152, "S4GUI in"=w10151) -> ("error out"=w10145:errorcluster, "S4GUI out"=w10144:refnum<class "S4GUI.lvclass">)  [unwired: 7 in]
          }
        }
      }
      event "Set Focus 2": Value Change {
        n4364 = event-data() -> ("NewVal"=w10162:bool)  [unwired: 1 in]
        n4365 = case shown="True" w10162 {
          tunnel: w10166 -> [w10168 w10177]
          tunnel: w10165 -> [w10167 w10176]
          tunnel: [w10167 w10175] -> w10164
          tunnel: [w10168 w10174] -> w10163
          frame False {
          }
          frame True {
            n4366 = call-dynamic "Read TelFocus.lvclass.vi"("error in (no error)"=w10176, "S4GUI in"=w10177) -> ("error out"=w10190:errorcluster, "TelFocus.lvclass"=w10191:refnum<class "TelFocus.lvclass">, "S4GUI out"=w10181:refnum<class "S4GUI.lvclass">)  [unwired: 7 in]
            n4367 = call-dynamic "Read SecMirror.lvclass.vi"("error in (no error)"=w10190, "TelFocus in"=w10191) -> ("error out"=w10171:errorcluster, "SecMirror.lvclass"=w10173:refnum<class "SecMirror.lvclass">, "TelFocus out"=w10184:refnum<class "TelFocus.lvclass">)  [unwired: 7 in]
            n4368 = call-dynamic "Write target.vi"("error in (no error)"=w10171, "target"="Target focus 2", "SecMirror in"=w10173) -> ("error out"=w10170:errorcluster, "SecMirror out"=w10172:refnum<class "SecMirror.lvclass">)  [unwired: 7 in]
            n4369 = call-dynamic "Read State Machine.vi"("error in (no error)"=w10170, "Device in"=w10172) -> ("error out"=w10188:errorcluster, "State Machine.lvclass"=w10189:refnum<class "State Machine.lvclass">, "Device out"=w10185:refnum<class "SecMirror.lvclass">)  [unwired: 7 in]
            n4370 = call "Next State.vi"("error in (no error)"=w10188, "New_State"=1, "State Machine in"=w10189) -> ("error out"=w10183:errorcluster, "State Machine out"=w10186:refnum<class "State Machine.lvclass">)  [unwired: 7 in]
            n4371 = call-dynamic "Write State Machine.vi"("error in (no error)"=w10183, "State Machine.lvclass"=w10186, "Device in"=w10185) -> ("error out"=w10179:errorcluster, "Device out"=w10178:refnum<class "SecMirror.lvclass">)  [unwired: 7 in]
            n4372 = call-dynamic "Write SecMirror.lvclass.vi"("error in (no error)"=w10179, "SecMirror.lvclass"=w10178, "TelFocus in"=w10184) -> ("error out"=w10180:errorcluster, "TelFocus out"=w10182:refnum<class "TelFocus.lvclass">)  [unwired: 7 in]
            n4373 = call-dynamic "Write TelFocus.lvclass.vi"("error in (no error)"=w10180, "TelFocus.lvclass"=w10182, "S4GUI in"=w10181) -> ("error out"=w10175:errorcluster, "S4GUI out"=w10174:refnum<class "S4GUI.lvclass">)  [unwired: 7 in]
          }
        }
      }
      event "Stop Focus", "Stop Focus 2": Value Change {
        n4374 = event-data() -> ("NewVal"=w10192:bool)  [unwired: 1 in]
        n4375 = case shown="True" w10192 {
          tunnel: w10196 -> [w10198 w10204]
          tunnel: w10195 -> [w10197 w10203]
          tunnel: [w10197 w10202] -> w10194
          tunnel: [w10198 w10201] -> w10193
          frame False {
          }
          frame True {
            n4376 = call-dynamic "Read TelFocus.lvclass.vi"("error in (no error)"=w10203, "S4GUI in"=w10204) -> ("error out"=w10217:errorcluster, "TelFocus.lvclass"=w10218:refnum<class "TelFocus.lvclass">, "S4GUI out"=w10208:refnum<class "S4GUI.lvclass">)  [unwired: 7 in]
            n4377 = call-dynamic "Read SecMirror.lvclass.vi"("error in (no error)"=w10217, "TelFocus in"=w10218) -> ("error out"=w10199:errorcluster, "SecMirror.lvclass"=w10200:refnum<class "SecMirror.lvclass">, "TelFocus out"=w10211:refnum<class "TelFocus.lvclass">)  [unwired: 7 in]
            n4378 = call-dynamic "Read State Machine.vi"("error in (no error)"=w10199, "Device in"=w10200) -> ("error out"=w10215:errorcluster, "State Machine.lvclass"=w10216:refnum<class "State Machine.lvclass">, "Device out"=w10212:refnum<class "SecMirror.lvclass">)  [unwired: 7 in]
            n4379 = call "Next State.vi"("error in (no error)"=w10215, "New_State"=10, "State Machine in"=w10216) -> ("error out"=w10210:errorcluster, "State Machine out"=w10213:refnum<class "State Machine.lvclass">)  [unwired: 7 in]
            n4380 = call-dynamic "Write State Machine.vi"("error in (no error)"=w10210, "State Machine.lvclass"=w10213, "Device in"=w10212) -> ("error out"=w10206:errorcluster, "Device out"=w10205:refnum<class "SecMirror.lvclass">)  [unwired: 7 in]
            n4381 = call-dynamic "Write SecMirror.lvclass.vi"("error in (no error)"=w10206, "SecMirror.lvclass"=w10205, "TelFocus in"=w10211) -> ("error out"=w10207:errorcluster, "TelFocus out"=w10209:refnum<class "TelFocus.lvclass">)  [unwired: 7 in]
            n4382 = call-dynamic "Write TelFocus.lvclass.vi"("error in (no error)"=w10207, "TelFocus.lvclass"=w10209, "S4GUI in"=w10208) -> ("error out"=w10202:errorcluster, "S4GUI out"=w10201:refnum<class "S4GUI.lvclass">)  [unwired: 7 in]
          }
        }
      }
      event "cooler ON 1": Value Change {
        n4383 = event-data() -> ("NewVal"=w10219:bool)  [unwired: 1 in]
        n4384 = case shown="True" w10219 {
          tunnel: [w10224 w10259] -> w10223
          tunnel: [w10225 w10258] -> w10222
          tunnel: w10221 -> [w10225 w10229]
          tunnel: w10220 -> [w10224 w10228]
          frame False {
          }
          frame True {
            w10227 = i16 1 items=["Cooler OFF", "Cooler ON"] ("Cooler ON/OFF")
            n4385 = Concatenate Strings("SET COOLER " ("User Event"), "ON ", "CLICKED - CH1" ("User Event")) -> (w10231:string)
            n4386 = call-dynamic "Write User Event.vi"("error in (no error)"=w10228, "User Event"=w10231, "S4GUI in"=w10229) -> ("error out"=w10232:errorcluster, "S4GUI out"=w10234:refnum<class "S4GUI.lvclass">)  [unwired: 7 in]
            n4387 = call-dynamic "Read AcquisitionA.vi"("error in (no error)"=w10232, "S4ACS_GUI in"=w10234) -> ("error out"=w10256:errorcluster, "Acquisition.lvclass"=w10257:refnum<class "Acquisition.lvclass">, "S4ACS_GUI out"=w10247:refnum<class "S4GUI.lvclass">)  [unwired: 7 in]
            n4388 = call-dynamic "Read Channel.vi"("error in (no error)"=w10256, "Acquisition in"=w10257) -> ("error out"=w10240:errorcluster, "Channel.lvclass"=w10244:refnum<class "Channel.lvclass">, "Acquisition out"=w10250:refnum<class "Acquisition.lvclass">)  [unwired: 7 in]
            n4389 = call-dynamic "Read Interface.vi"("error in (no error)"=w10240, "Channel in"=w10244) -> ("error out"=w10235:errorcluster, "Interface.lvclass"=w10236:refnum<class "Interface.lvclass">, "Channel out"=w10243:refnum<class "Channel.lvclass">)  [unwired: 7 in]
            n4390 = call-dynamic "Write Cooler ON_OFF.vi"("error in (no error)"=w10235, "Cooler ON/OFF"=w10227, "Interface in"=w10236) -> ("error out"=w10239:errorcluster, "Interface out"=w10241:refnum<class "Interface.lvclass">)  [unwired: 7 in]
            n4391 = call-dynamic "Write Interface.vi"("error in (no error)"=w10239, "Interface.lvclass"=w10241, "Channel in"=w10243) -> ("error out"=w10238:errorcluster, "Channel out"=w10242:refnum<class "Channel.lvclass">)  [unwired: 7 in]
            n4392 = call-dynamic "Read State Machine.vi"("error in (no error)"=w10238, "Device in"=w10242) -> ("error out"=w10254:errorcluster, "State Machine.lvclass"=w10255:refnum<class "State Machine.lvclass">, "Device out"=w10251:refnum<class "Channel.lvclass">)  [unwired: 7 in]
            n4393 = call "Next State.vi"("error in (no error)"=w10254, "New_State"=u32 30, "State Machine in"=w10255) -> ("error out"=w10249:errorcluster, "State Machine out"=w10252:refnum<class "State Machine.lvclass">)  [unwired: 7 in]
            n4394 = call-dynamic "Write State Machine.vi"("error in (no error)"=w10249, "State Machine.lvclass"=w10252, "Device in"=w10251) -> ("error out"=w10245:errorcluster, "Device out"=w10237:refnum<class "Channel.lvclass">)  [unwired: 7 in]
            n4395 = call-dynamic "Write Channel.vi"("error in (no error)"=w10245, "Channel.lvclass"=w10237, "Acquisition in"=w10250) -> ("error out"=w10246:errorcluster, "Acquisition out"=w10248:refnum<class "Acquisition.lvclass">)  [unwired: 7 in]
            n4396 = call-dynamic "Write AcquisitionA.vi"("error in (no error)"=w10246, "Acquisition.lvclass"=w10248, "S4ACS_GUI in"=w10247) -> ("error out"=w10259:errorcluster, "S4ACS_GUI out"=w10258:refnum<class "S4GUI.lvclass">)  [unwired: 7 in]
          }
        }
      }
      event "cooler ON 2": Value Change {
        n4397 = event-data() -> ("NewVal"=w10260:bool)  [unwired: 1 in]
        n4398 = case shown="True" w10260 {
          tunnel: [w10265 w10300] -> w10264
          tunnel: [w10266 w10299] -> w10263
          tunnel: w10262 -> [w10266 w10270]
          tunnel: w10261 -> [w10265 w10269]
          frame False {
          }
          frame True {
            w10268 = i16 1 items=["Cooler OFF", "Cooler ON"] ("Cooler ON/OFF")
            n4399 = Concatenate Strings("SET COOLER " ("User Event"), "ON ", "CLICKED - CH2" ("User Event")) -> (w10272:string)
            n4400 = call-dynamic "Write User Event.vi"("error in (no error)"=w10269, "User Event"=w10272, "S4GUI in"=w10270) -> ("error out"=w10273:errorcluster, "S4GUI out"=w10275:refnum<class "S4GUI.lvclass">)  [unwired: 7 in]
            n4401 = call "Read AcquisitionB.vi"("error in (no error)"=w10273, "S4ACS_GUI in"=w10275) -> ("error out"=w10297:errorcluster, "Acquisition.lvclass"=w10298:refnum<class "Acquisition.lvclass">, "S4ACS_GUI out"=w10288:refnum<class "S4GUI.lvclass">)  [unwired: 7 in]
            n4402 = call-dynamic "Read Channel.vi"("error in (no error)"=w10297, "Acquisition in"=w10298) -> ("error out"=w10281:errorcluster, "Channel.lvclass"=w10285:refnum<class "Channel.lvclass">, "Acquisition out"=w10291:refnum<class "Acquisition.lvclass">)  [unwired: 7 in]
            n4403 = call-dynamic "Read Interface.vi"("error in (no error)"=w10281, "Channel in"=w10285) -> ("error out"=w10276:errorcluster, "Interface.lvclass"=w10277:refnum<class "Interface.lvclass">, "Channel out"=w10284:refnum<class "Channel.lvclass">)  [unwired: 7 in]
            n4404 = call-dynamic "Write Cooler ON_OFF.vi"("error in (no error)"=w10276, "Cooler ON/OFF"=w10268, "Interface in"=w10277) -> ("error out"=w10280:errorcluster, "Interface out"=w10282:refnum<class "Interface.lvclass">)  [unwired: 7 in]
            n4405 = call-dynamic "Write Interface.vi"("error in (no error)"=w10280, "Interface.lvclass"=w10282, "Channel in"=w10284) -> ("error out"=w10279:errorcluster, "Channel out"=w10283:refnum<class "Channel.lvclass">)  [unwired: 7 in]
            n4406 = call-dynamic "Read State Machine.vi"("error in (no error)"=w10279, "Device in"=w10283) -> ("error out"=w10295:errorcluster, "State Machine.lvclass"=w10296:refnum<class "State Machine.lvclass">, "Device out"=w10292:refnum<class "Channel.lvclass">)  [unwired: 7 in]
            n4407 = call "Next State.vi"("error in (no error)"=w10295, "New_State"=u32 30, "State Machine in"=w10296) -> ("error out"=w10290:errorcluster, "State Machine out"=w10293:refnum<class "State Machine.lvclass">)  [unwired: 7 in]
            n4408 = call-dynamic "Write State Machine.vi"("error in (no error)"=w10290, "State Machine.lvclass"=w10293, "Device in"=w10292) -> ("error out"=w10286:errorcluster, "Device out"=w10278:refnum<class "Channel.lvclass">)  [unwired: 7 in]
            n4409 = call-dynamic "Write Channel.vi"("error in (no error)"=w10286, "Channel.lvclass"=w10278, "Acquisition in"=w10291) -> ("error out"=w10287:errorcluster, "Acquisition out"=w10289:refnum<class "Acquisition.lvclass">)  [unwired: 7 in]
            n4410 = call "Write AcquisitionB.vi"("error in (no error)"=w10287, "Acquisition.lvclass"=w10289, "S4ACS_GUI in"=w10288) -> ("error out"=w10300:errorcluster, "S4ACS_GUI out"=w10299:refnum<class "S4GUI.lvclass">)  [unwired: 7 in]
          }
        }
      }
      event "cooler ON 3": Value Change {
        n4411 = event-data() -> ("NewVal"=w10301:bool)  [unwired: 1 in]
        n4412 = case shown="True" w10301 {
          tunnel: [w10306 w10341] -> w10305
          tunnel: [w10307 w10340] -> w10304
          tunnel: w10303 -> [w10307 w10311]
          tunnel: w10302 -> [w10306 w10310]
          frame False {
          }
          frame True {
            w10309 = i16 1 items=["Cooler OFF", "Cooler ON"] ("Cooler ON/OFF")
            n4413 = Concatenate Strings("SET COOLER " ("User Event"), "ON ", "CLICKED - CH3" ("User Event")) -> (w10313:string)
            n4414 = call-dynamic "Write User Event.vi"("error in (no error)"=w10310, "User Event"=w10313, "S4GUI in"=w10311) -> ("error out"=w10314:errorcluster, "S4GUI out"=w10316:refnum<class "S4GUI.lvclass">)  [unwired: 7 in]
            n4415 = call-dynamic "Read AcquisitionC.vi"("error in (no error)"=w10314, "S4ACS_GUI in"=w10316) -> ("error out"=w10338:errorcluster, "Acquisition.lvclass"=w10339:refnum<class "Acquisition.lvclass">, "S4ACS_GUI out"=w10329:refnum<class "S4GUI.lvclass">)  [unwired: 7 in]
            n4416 = call-dynamic "Read Channel.vi"("error in (no error)"=w10338, "Acquisition in"=w10339) -> ("error out"=w10322:errorcluster, "Channel.lvclass"=w10326:refnum<class "Channel.lvclass">, "Acquisition out"=w10332:refnum<class "Acquisition.lvclass">)  [unwired: 7 in]
            n4417 = call-dynamic "Read Interface.vi"("error in (no error)"=w10322, "Channel in"=w10326) -> ("error out"=w10317:errorcluster, "Interface.lvclass"=w10318:refnum<class "Interface.lvclass">, "Channel out"=w10325:refnum<class "Channel.lvclass">)  [unwired: 7 in]
            n4418 = call-dynamic "Write Cooler ON_OFF.vi"("error in (no error)"=w10317, "Cooler ON/OFF"=w10309, "Interface in"=w10318) -> ("error out"=w10321:errorcluster, "Interface out"=w10323:refnum<class "Interface.lvclass">)  [unwired: 7 in]
            n4419 = call-dynamic "Write Interface.vi"("error in (no error)"=w10321, "Interface.lvclass"=w10323, "Channel in"=w10325) -> ("error out"=w10320:errorcluster, "Channel out"=w10324:refnum<class "Channel.lvclass">)  [unwired: 7 in]
            n4420 = call-dynamic "Read State Machine.vi"("error in (no error)"=w10320, "Device in"=w10324) -> ("error out"=w10336:errorcluster, "State Machine.lvclass"=w10337:refnum<class "State Machine.lvclass">, "Device out"=w10333:refnum<class "Channel.lvclass">)  [unwired: 7 in]
            n4421 = call "Next State.vi"("error in (no error)"=w10336, "New_State"=u32 30, "State Machine in"=w10337) -> ("error out"=w10331:errorcluster, "State Machine out"=w10334:refnum<class "State Machine.lvclass">)  [unwired: 7 in]
